vi "Write To String Delimiter.vi"(8 "error in (no error)":errorcluster, 10 "Delimiter":string, 11 "Abs_Boolean_1D in":refnum<class "Abs_Boolean_1D.lvclass">) -> (0 "error out":errorcluster, 3 "Abs_Boolean_1D out":refnum<class "Abs_Boolean_1D.lvclass">)   [LabVIEW 2021, in "Abs_Boolean_1D.lvclass"]
uses:
  Abs_Boolean_1D.lvclass
  Abs_Boolean_1D.lvclass/Abs_Boolean_1D.ctl
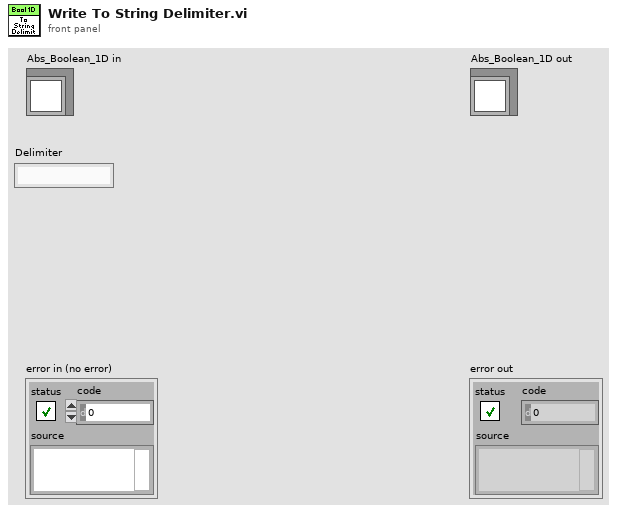
[diagram p1: front panel]
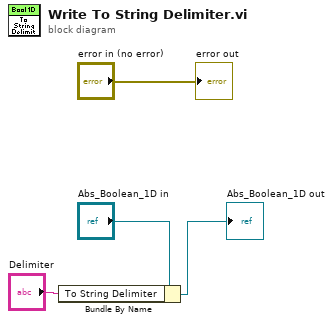
[diagram p0: block diagram]
diagram:
  n1 = Bundle By Name(cluster="Abs_Boolean_1D in", "To String Delimiter"="Delimiter") -> (→"Abs_Boolean_1D out":refnum<class "Abs_Boolean_1D.lvclass">)
  "error out" <- "error in (no error)"
